vi "Get SSR Status - All.vi"(0 "reference in":refnum<class "SSR.lvclass">, 5 "error in (no error)":errorcluster) -> (14 "reference out":refnum<class "SSR.lvclass">, 17 "All DO Status":bool[](array[boolean]), 19 "error out":errorcluster)   [LabVIEW 2017, in "SSR.lvclass"]
uses:
  SSR.lvclass
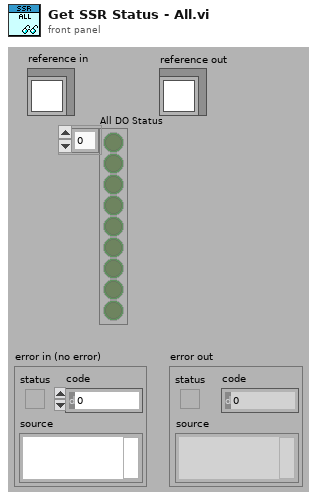
[diagram p1: front panel]
types:
  T1 = typedef "SSR.lvclass/ObjectAttributes.ctl" = cluster{"SSR Task":refnum<k21>, "SSR On/Off Status":bool, "Number of SSR Modules":u32, "Number of Total SSR Channels":u32, "SSR Module Names (NI-Max Name)":string[], "Number of Channels Per SSR Module":i32[], "SSR Status":bool[], "SSR Status to Set":bool[], "SSR VI Reference":refnum<vi>}
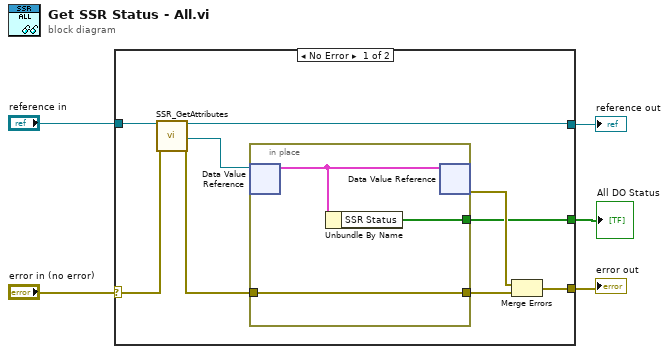
[diagram p0: block diagram]
diagram:
  n1 = case shown="No Error" "error in (no error)" {
    selector: "error in (no error)" -> [w13 w19]
    tunnel: [w10 w19] -> w4
    tunnel: [w11 w18] -> w2
    tunnel: "reference in" -> [w14 w18]
    tunnel: [w6 _] -> w1
    frame No Error {
      n2 = call "SSR_GetAttributes.vi"("reference in"=w14, "error in (no error)"=w13) -> ("reference out"=w11:refnum<class "SSR.lvclass">, "DataRef"=w9:refnum<data-value>, "error out"=w8:errorcluster)  [unwired: 14 in, 1 out]
      n3 = in-place {
        in-place-border: w8 -> [w17]
        in-place-border: [w17] -> w7
        in-place-border: [w15] -> w6
        n4 = in-place-dvr #1(w9) -> (w16:T1)  [unwired: 1 out]
        n5 = Unbundle By Name(w16) -> ("SSR Status"=w15:bool[])
        n6 = in-place-dvr #1(w16) -> (w12:errorcluster)  [unwired: 1 out]
      }
      n7 = Merge Errors(w12, w7) -> (w10:errorcluster)
    }
    frame Error {
    }
  }
  "error out" <- w4
  "reference out" <- w2
  "All DO Status" <- w1
